vi "Ramp_Advanced_Bias.vi"(0 "Sampling frequency (20000) / Hz":dbl=20000.0, 1 "Bias Modulation Frequency (100) / Hz":dbl=100.0, 2 "PM wave shape":dbl(ring) items=["triangle", "square", "sine"], 3 "# Steps (10)":i32=10, 4 "Ramp Time (1) / s":dbl=1.0, 5 "Error In":errorcluster, 6 "Measurement Type / bias":u16(ring) items=["Piezo Hold", "Square Bias", "Sine Bias", "Triangle Bias", "IV", "PM", "IV - Polarity Sweep", "CV - 2 Terminal", "Pre/Post Pulse IVs"], 7 "DC Bias (0.2) / V":dbl=0.2, 8 "DC time (0.02) / s":dbl=0.02, 9 "Pulse Bias / V":dbl=2.0, 10 "Piezo Modulation freq.":dbl, 11 "Step Height (1) / nm":dbl=1.0, 12 "PM compression legnth / nm":dbl, 13 "Bias Ramp Amplitude (1) / V":dbl=1.0) -> (14 "Piezo Out / nm":dbl[](array[numeric]), 15 "Waveform Graph":dbl[][](graph), 17 "Bias Ramp Out / V":dbl[](array[numeric]), 19 "Error Out":errorcluster)   [LabVIEW 2025]
panel:
  out "Waveform Graph 2":dbl[](graph)
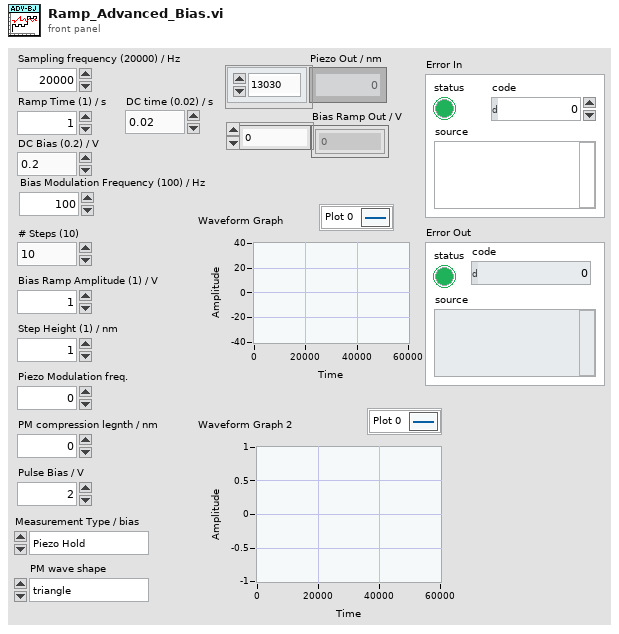
[diagram p1: front panel]
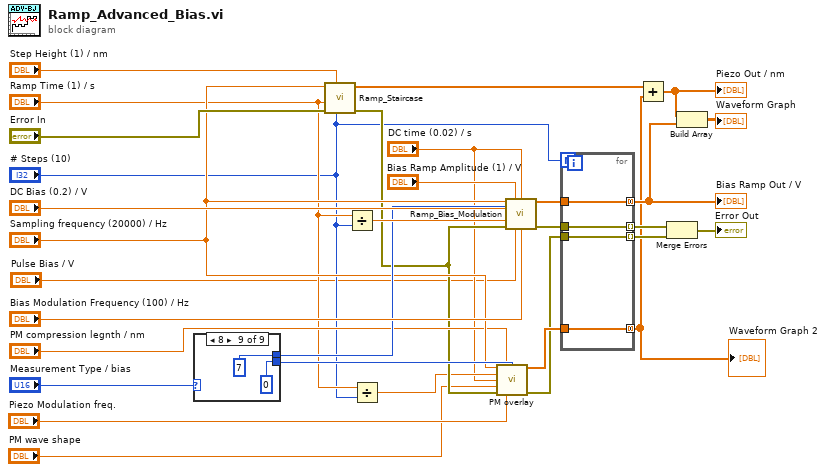
[diagram p0: block diagram]
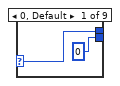
[diagram p2: hidden frame]
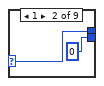
[diagram p3: hidden frame]
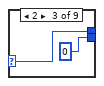
[diagram p4: hidden frame]
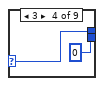
[diagram p5: hidden frame]
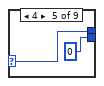
[diagram p6: hidden frame]
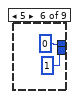
[diagram p7: hidden frame]
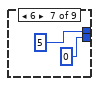
[diagram p8: hidden frame]
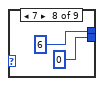
[diagram p9: hidden frame]
diagram:
  n1 = case shown="8" "Measurement Type / bias" {
    selector: "Measurement Type / bias" -> [w33 w35 w36 w38 w41 _ _ _ _]
    tunnel: [w33 w35 w36 w38 w41 0 5 ("Measurement Type / bias") 6 ("Measurement Type / bias") 7 ("Measurement Type / bias")] -> w22
    tunnel: [0 0 0 0 0 1 0 0 0] -> w21
    frame 0, Default {
    }
    frame 1 {
    }
    frame 2 {
    }
    frame 3 {
    }
    frame 4 {
    }
    frame 5 {
    }
    frame 6 {
    }
    frame 7 {
    }
    frame 8 {
    }
  }
  n2 = call "Ramp_Staircase.vi"("# Steps (10)"="# Steps (10)", "Step Height (1) / nm"="Step Height (1) / nm", "Error In"="Error In", "Ramp Time (1) / s"="Ramp Time (1) / s", "Acquisition Rate (20000) / Hz"="Sampling frequency (20000) / Hz") -> ("Error Out"=w15:errorcluster, "Piezo Out / nm"=w9:dbl[])  [unwired: 4 in]
  n3 = Divide(x="Ramp Time (1) / s", y="# Steps (10)") -> (x/y=w31:dbl)
  n4 = Divide(x="Ramp Time (1) / s", y="# Steps (10)") -> (x/y=w3:dbl)
  n5 = call "PM overlay.vi"("Sampling frequency (20000) / Hz"="Sampling frequency (20000) / Hz", "Ramp Amplitude (1) / nm"="PM compression legnth / nm", "Text Ring"=w21, "Ramp Length (0.1) / s"=w3, "Lead time (0.01) / s"="DC time (0.02) / s", "PM wave shape"="PM wave shape", "Error In"=w15, "Modulation Frequency (10) / Hz"="Piezo Modulation freq.") -> ("PM wave overlay"=w19:dbl[], "Error Out"=w11:errorcluster)  [unwired: 6 in]
  n6 = call "Ramp_Bias_Modulation.vi"("Sampling frequency (20000) / Hz"="Sampling frequency (20000) / Hz", "Ramp Amplitude (1) / V"="Bias Ramp Amplitude (1) / V", "DC time (0.02) / s"="DC time (0.02) / s", "Text Ring"=w22, "DC Bias (0.2) / V"="DC Bias (0.2) / V", "Ramp Length (0.1) / s"=w31, "Error In"=w15, "Pulse bias /V"="Pulse Bias / V", "Modulation Frequency (100) / Hz"="Bias Modulation Frequency (100) / Hz") -> ("Bias Ramp Out / V"=w25:dbl[], "Error Out"=w13:errorcluster)  [unwired: 5 in]
  n7 = for {
    N: "# Steps (10)" -> [_]
    tunnel: w25 -> [w53]
    tunnel: [w53] -> w24 mode=concatenating
    tunnel: w19 -> [w52]
    tunnel: [w52] -> w7 mode=concatenating
    tunnel: w13 -> [w51]
    tunnel: [w51] -> w12 mode=indexing
    tunnel: w11 -> [w50]
    tunnel: [w50] -> w10 mode=indexing
  }
  "Bias Ramp Out / V" <- w24
  "Waveform Graph 2" <- w7
  n8 = Add(x=w9, y=w7) -> (x+y=w8:dbl[])
  "Piezo Out / nm" <- w8
  n9 = Merge Errors(w12, w10) -> (→"Error Out":errorcluster)
  n10 = Build Array(w8, w24) -> (→"Waveform Graph":dbl[][])
